vi "PSPara_Para Setting Operation.vi"(7 "Operation":enum16{"Set Value", "Get Value", "Initialize"}(ring)=enum."Get Value", 9 "error in":errorcluster, 10 "_Para":T1={"Timing"={"SampleRate"=1000}, "SavePara"={"FlowDiskMode"=0, "SelectMode"=0, "FolderPath"=path "", "Filename"="演示", "FileNote"="演示", "AutoInterval"=0, "Template"=path ""}, "ConfigDS Path*"=path "", "Tdms Ref*"=refnum} {"SavePara"."SelectMode" items=["手动挑点", "自动挑点"]; "SavePara"."FlowDiskMode" items=["不存储", "连续存储"]; "Timing"."SampleRate" items=["1S/s"=1, "2S/s"=2, "5S/s"=5, "10S/s"=10, "20S/s"=20, "50S/s"=50, "100S/s"=100, "200S/s"=200, "500S/s"=500, "1KS/s"=1000, "2KS/s"=2000, "5KS/s"=5000, "10KS/s"=10000, "20KS/s"=20000, "50KS/s"=50000, "100KS/s"=100000, "200KS/s"=200000]}) -> (1 "error out":errorcluster, 2 "_Para":T1={"Timing"={"SampleRate"=1000}, "SavePara"={"FlowDiskMode"=0, "SelectMode"=0, "FolderPath"=path "", "Filename"="演示", "FileNote"="演示", "AutoInterval"=0, "Template"=path ""}, "ConfigDS Path*"=path "", "Tdms Ref*"=refnum} {"SavePara"."SelectMode" items=["手动挑点", "自动挑点"]; "SavePara"."FlowDiskMode" items=["不存储", "连续存储"]; "Timing"."SampleRate" items=["1S/s"=1, "2S/s"=2, "5S/s"=5, "10S/s"=10, "20S/s"=20, "50S/s"=50, "100S/s"=100, "200S/s"=200, "500S/s"=500, "1KS/s"=1000, "2KS/s"=2000, "5KS/s"=5000, "10KS/s"=10000, "20KS/s"=20000, "50KS/s"=50000, "100KS/s"=100000, "200KS/s"=200000]})   [LabVIEW 2016]
doc: "设定系统存储参数"
uses:
  Controls/Global para Config.ctl
  File Save Mode.ctl
  Select Point Mode.ctl
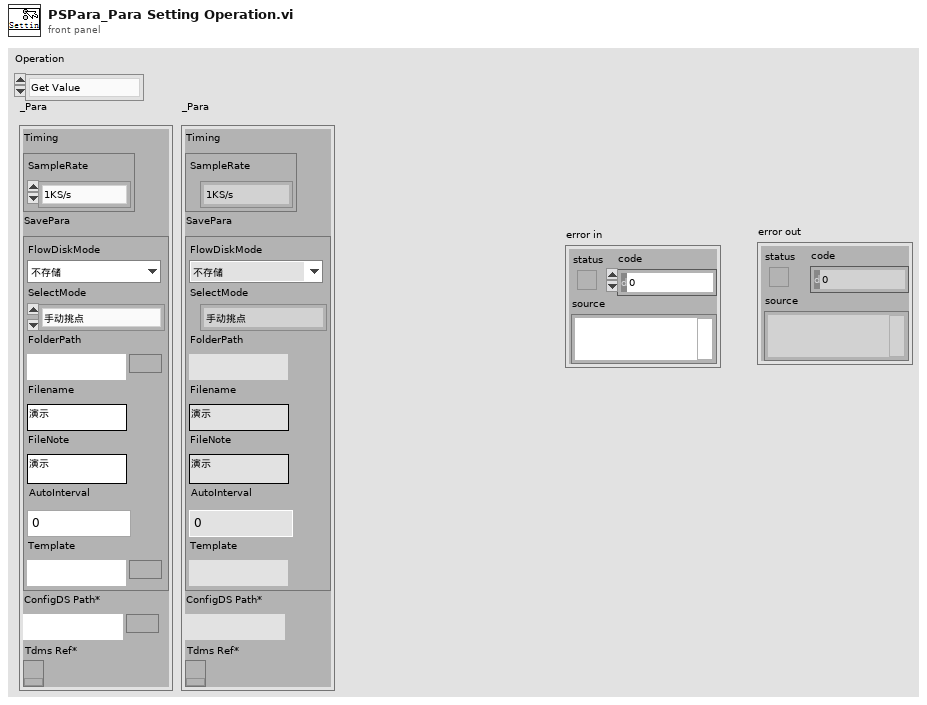
[diagram p1: front panel]
types:
  T1 = typedef "Global para Config.ctl" = cluster{"Timing":cluster{"SampleRate":i32}, "SavePara":cluster{"FlowDiskMode":T2, "SelectMode":T3, "FolderPath":path, "Filename":string, "FileNote":string, "AutoInterval":i32, "Template":path}, "ConfigDS Path*":path, "Tdms Ref*":refnum<k34>}
  T2 = typedef "File Save Mode.ctl" = i32
  T3 = typedef "Select Point Mode.ctl" = i32
  T4 = cluster{"DfltDataFolder":path, "ParaFolder":path, "SysCfg":path, "CHdef":path, "ModCfg":path, "DT Folder":path, "ErrorLog":path, "HBMlic":path}
  T5 = cluster{"Folder":path, "FileName":string, "FileNote":string, "AutoInterval":i32}
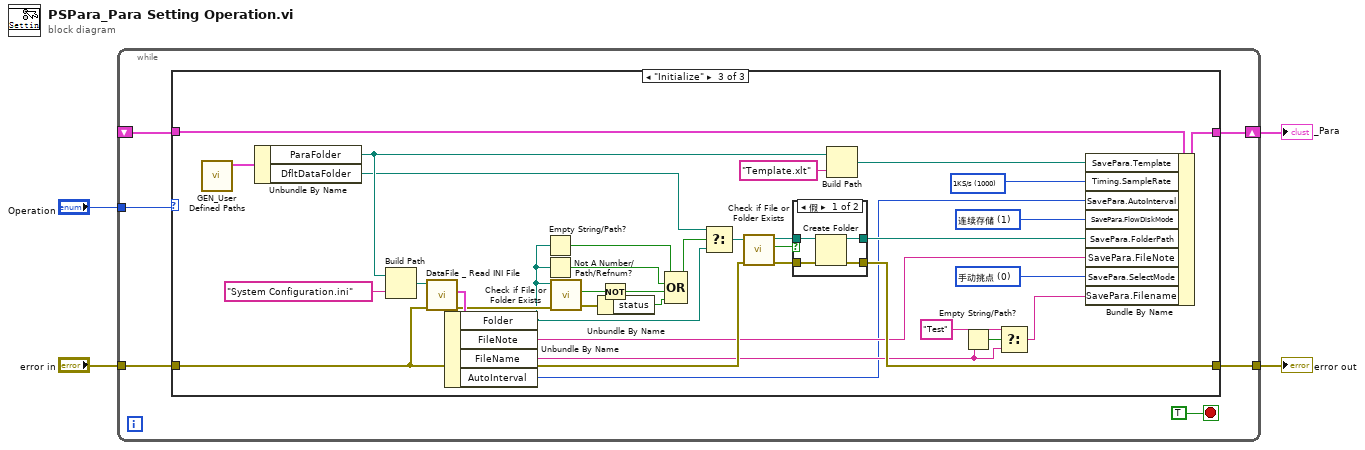
[diagram p0: block diagram]
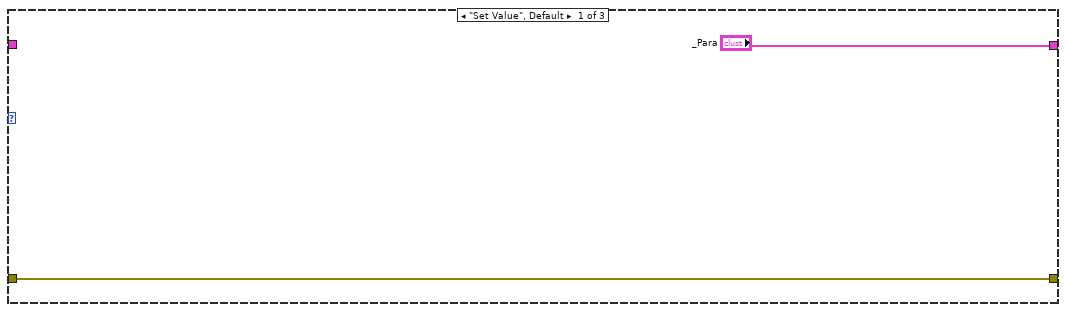
[diagram p2: hidden frame]
diagram:
  n1 = while {
    tunnel: "Operation" -> [w9]
    shift-right: [w8] -> w1
    shift-left: _ -> [w7]
    tunnel: "error in" -> [w6]
    tunnel: [w5] -> w2
    stop <- TRUE stop-if-true
    n2 = case shown="\"Initialize\"" w9 {
      tunnel: ["_Para" w14 w48] -> w8
      tunnel: w7 -> [_ w14 w49]
      tunnel: w6 -> [w11 w13 w24]
      tunnel: [w11 w13 w41] -> w5
      frame "Set Value", Default {
      }
      frame "Get Value" {
      }
      frame "Initialize" {
        w40 = T3 0 items=["手动挑点", "自动挑点"] ("SavePara.SelectPointMode")
        w46 = 1000 items=["1S/s"=1, "2S/s"=2, "5S/s"=5, "10S/s"=10, "20S/s"=20, "50S/s"=50, "100S/s"=100, "200S/s"=200, "500S/s"=500, "1KS/s"=1000, "2KS/s"=2000, "5KS/s"=5000, "10KS/s"=10000, "20KS/s"=20000, "50KS/s"=50000, "100KS/s"=100000, "200KS/s"=200000] ("SampleRate")
        w47 = T2 1 items=["不存储", "连续存储"] ("Save Mode")
        n3 = call "GEN_User Defined Paths.vi"() -> ("UserDefinedPath"=w45:T4)  [unwired: 11 in]
        n4 = Unbundle By Name(w45) -> ("ParaFolder"=w28:path, "DfltDataFolder"=w26:path)
        n5 = Build Path(base path=w28, name or relative path="System Configuration.ini") -> (appended path=w35:path)
        n6 = call "DataFile _ Read INI File.vi"("error in"=w24, "configuration file path"=w35) -> ("error out"=w33:errorcluster, "value"=w34:T5)  [unwired: 8 in]
        n7 = Unbundle By Name(w34) -> ("Folder"=w18:path, "FileNote"=w16:string, "FileName"=w22:string, "AutoInterval"=w15:i32)
        n8 = Empty String/Path?(string/path=w18) -> (empty?=w17:bool)
        n9 = Not A Number/Path/Refnum?(number/path/refnum=w18) -> (NaN/Path/Refnum?=w19:bool)
        n10 = call <vilib>:"Check if File or Folder Exists.vi"("error in (no error)"=w33, "path"=w18) -> ("error out"=w31:errorcluster, "file or folder exists?"=w32:bool)  [unwired: 7 in, 1 out]
        n11 = Unbundle By Name(w31) -> ("status"=w30:bool)
        n12 = Not(x=w32) -> (.not. x?=w29:bool)
        n13 = Compound Arithmetic op=OR ("复合运算")(w17, w19, w29, w30) -> (w27:bool)
        n14 = Select(t=w26, s=w27, f=w18) -> (s? t:f=w25:path)
        n15 = call <vilib>:"Check if File or Folder Exists.vi"("error in (no error)"=w24, "path"=w25) -> ("error out"=w43:errorcluster, "file or folder exists?"=w44:bool, "dup path"=w42:path)  [unwired: 7 in]
        n16 = case shown="假" w44 {
          tunnel: w43 -> [w52 w54]
          tunnel: w42 -> [w53 w55]
          tunnel: [w51 w55] -> w39
          tunnel: [w50 w54] -> w41
          frame False {
            n17 = Create Folder(path (use dialog)=w53, error in=w52) -> (created path=w51:path, error out=w50:errorcluster)  [unwired: 1 in, 1 out]
          }
          frame True {
          }
        }
        n18 = Build Path(base path=w28, name or relative path="Template.xlt") -> (appended path=w37:path)
        n19 = Empty String/Path?(string/path=w22) -> (empty?=w23:bool)
        n20 = Select(t="Test", s=w23, f=w22) -> (s? t:f=w20:string)
        n21 = Bundle By Name(cluster=w49, "SavePara.Template"=w37, "Timing.SampleRate"=w46, "SavePara.AutoInterval"=w15, "SavePara.FlowDiskMode"=w47, "SavePara.FolderPath"=w39, "SavePara.FileNote"=w16, "SavePara.SelectMode"=w40, "SavePara.Filename"=w20) -> (w48:T1)
      }
    }
  }
  "error out" <- w2
  "_Para" <- w1
